vi "A180648.vi"() -> ()   [LabVIEW 2020]
panel:
  in  "工位二动态曲线":refnum<vi>
  in  "工位一动态曲线":refnum<vi>
  in  "工位二复检曲线":refnum<vi>
  in  "工位一复检曲线":refnum<vi>
  in  "CAN_CYCLE":T1(array[cluster]) {"周期(ms)" min=1 format="%d ms"; "ID" format="0x%x"}
  in  "功能试验参数":T2
  in  "逆向空载试验参数":T3
  in  "试验结果":refnum<vi>
  in  "试验条件":refnum<vi>
  out "检测条件":string[][][](array[string])
  in  "当前检测项":T4(ring)=enum."力特性"
  out "检测结果":string[][][](array[string])
  in  "力特性":T5
  in  "空载":T6
  in  "逆向空载曲线":refnum<vi>
  in  "振动NVH曲线":refnum<vi>
  in  "电流特性曲线":refnum<vi>
  in  "LED-逆向空载":refnum<vi>
  in  "LED-振动NVH":refnum<vi>
  in  "LED-电流特性":refnum<vi>
  in  "功能":T7
  in  "传感器特性曲线":refnum<vi>
  in  "LED-传感器特性":refnum<vi>
  in  "LED-力特性":refnum<vi>
  in  "LED-功能":refnum<vi>
  in  "LED-空载":refnum<vi>
  in  "试验项":T8(tab)
  in  "空载曲线":refnum<vi>
  in  "力特性曲线":refnum<vi>
  in  "功能曲线":refnum<vi>
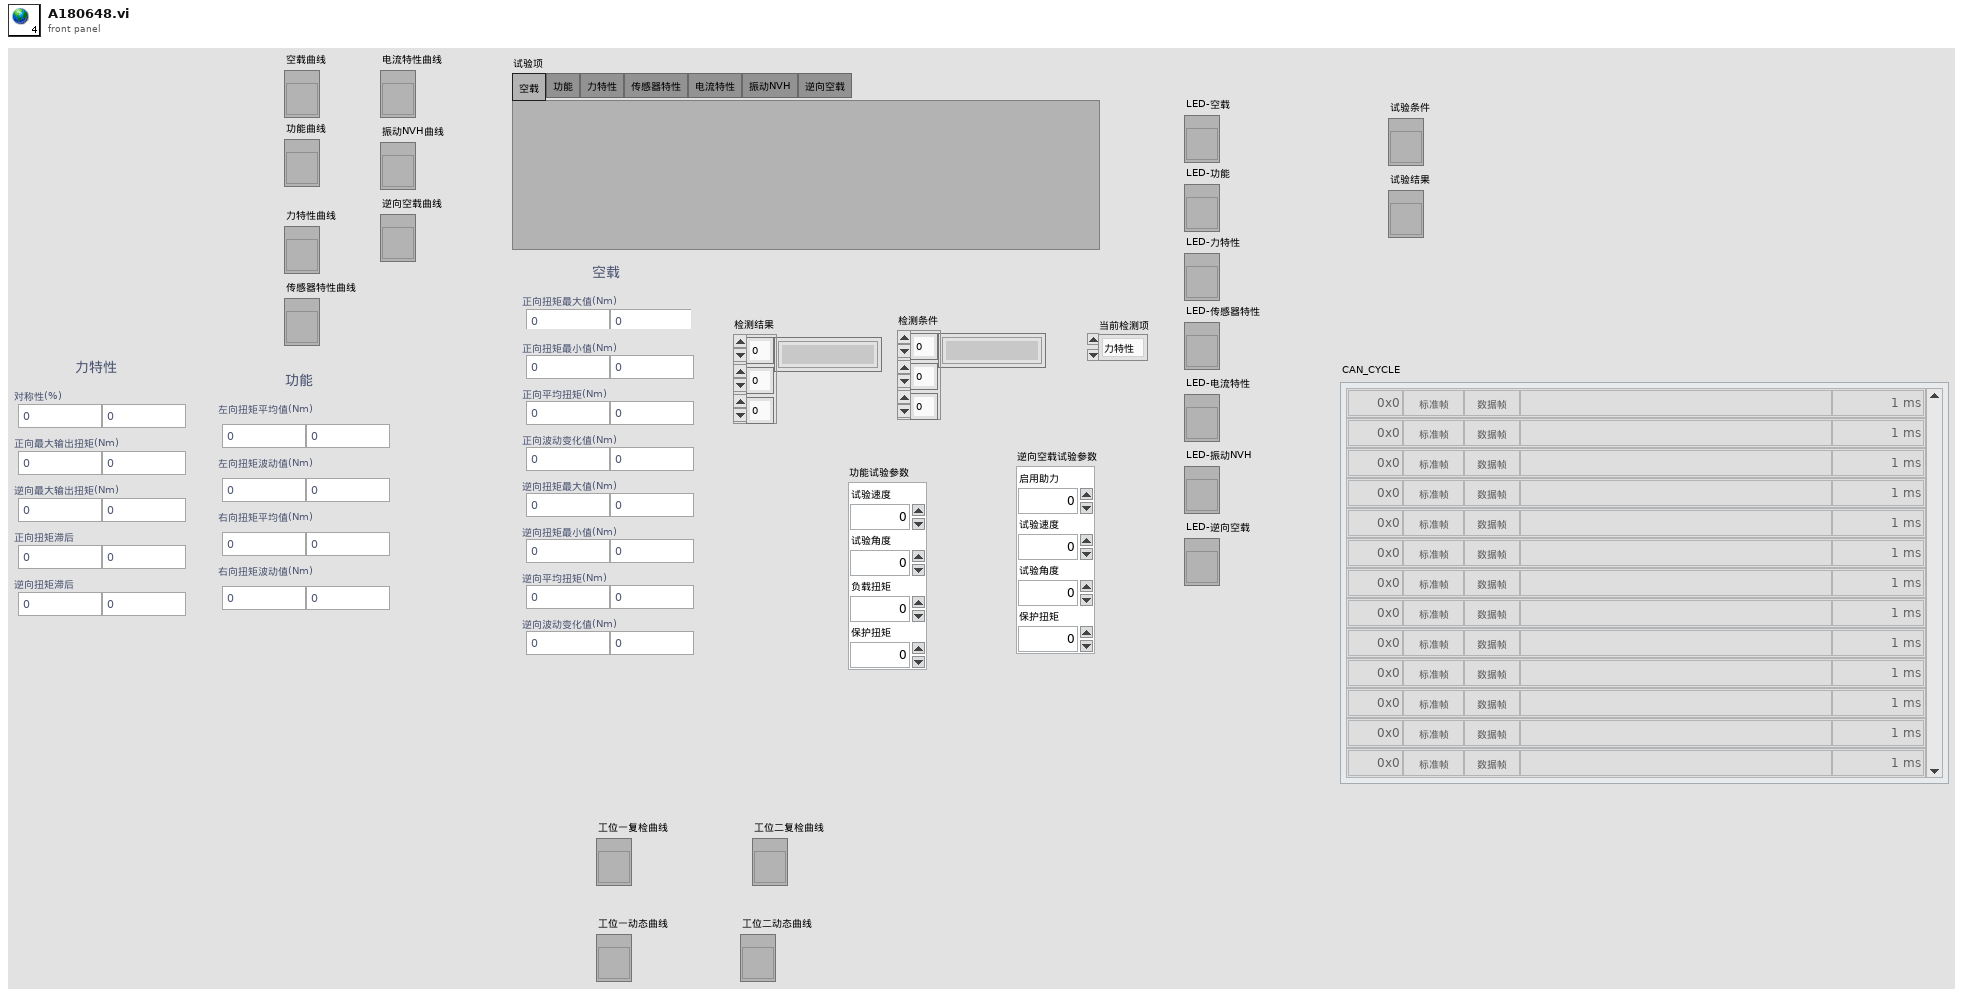
[diagram p1: front panel]
types:
  T1 = cluster{"ID":u32, "帧类型":enum8{"标准帧", "扩展帧"}, "帧格式":enum16{"数据帧", "远程帧"}, "帧数据":string, "周期(ms)":u32}[]
  T2 = cluster{"试验速度":dbl, "试验角度":dbl, "负载扭矩":dbl, "保护扭矩":dbl}
  T3 = cluster{"启用助力":dbl, "试验速度":dbl, "试验角度":dbl, "保护扭矩":dbl}
  T4 = enum32{"空载", "功能", "力特性", "传感器特性", "电流特性", "振动NVH", "逆向空载", "完成"}
  T5 = cluster{"对称性(%)":cluster{"下限":dbl, "上限":dbl}, "正向最大输出扭矩(Nm)":cluster{"下限":dbl, "上限":dbl}, "逆向最大输出扭矩(Nm)":cluster{"下限":dbl, "上限":dbl}, "正向扭矩滞后":cluster{"下限":dbl, "上限":dbl}, "逆向扭矩滞后":cluster{"下限":dbl, "上限":dbl}}
  T6 = cluster{"正向扭矩最大值(Nm)":cluster{"下限":dbl, "上限":dbl}, "正向扭矩最小值(Nm)":cluster{"下限":dbl, "上限":dbl}, "正向平均扭矩(Nm)":cluster{"下限":dbl, "上限":dbl}, "正向波动变化值(Nm)":cluster{"下限":dbl, "上限":dbl}, "逆向扭矩最大值(Nm)":cluster{"下限":dbl, "上限":dbl}, "逆向扭矩最小值(Nm)":cluster{"下限":dbl, "上限":dbl}, "逆向平均扭矩(Nm)":cluster{"下限":dbl, "上限":dbl}, "逆向波动变化值(Nm)":cluster{"下限":dbl, "上限":dbl}}
  T7 = cluster{"左向扭矩平均值(Nm)":cluster{"下限":dbl, "上限":dbl}, "左向扭矩波动值(Nm)":cluster{"下限":dbl, "上限":dbl}, "右向扭矩平均值(Nm)":cluster{"下限":dbl, "上限":dbl}, "右向扭矩波动值(Nm)":cluster{"下限":dbl, "上限":dbl}}
  T8 = enum32{"空载", "功能", "力特性", "传感器特性", "电流特性", "振动NVH", "逆向空载"}
diagram:
